vi "Configure.vi"(8 "error in":errorcluster, 10 "name":string, 11 "cPAS in":refnum<class "cPAS.lvclass">) -> (0 "error out":errorcluster, 3 "cPAS out":refnum<class "cPAS.lvclass">)   [LabVIEW 2015, in "cPAS.lvclass"]
doc: "Configure the Instrument object. The default behavior is to provide a name and define a command enqueuer."
uses:
  cPAS.lvclass
  Data/cPAS Data.lvclass
  Data/cPAS Cell Data/cPAS Cell Data.lvclass
  Reusable/PAS/Data/Main/Write CellData.vi
  Reusable/PAS/Main/Write Data.vi
  Reusable/PAS/Main/PAS.lvclass
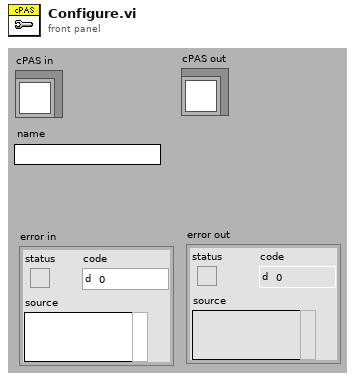
[diagram p1: front panel]
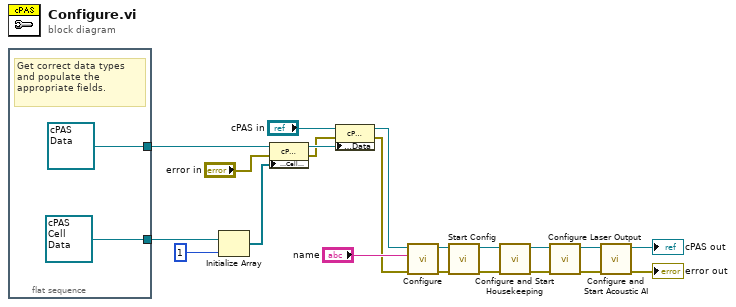
[diagram p0: block diagram]
diagram:
  n1 = flat-sequence {
    tunnel: [refnum<class "cPAS Data.lvclass"> refnum ("cPAS Data")] -> w10
    tunnel: [refnum<class "cPAS Cell Data.lvclass"> refnum ("cPAS Cell")] -> w9
    frame #0 {
      # "Get correct data types and populate the appropriate fields."
    }
  }
  n2 = Initialize Array(w9, 1 ("dimension size")) -> (w7:refnum<class "cPAS Cell Data.lvclass">[])
  n3 = property class="cPAS Data"(reference=w10, error in="error in", "Data Access:Cell Data"=w7) -> (reference out=w4:refnum<class "cPAS Data.lvclass">, error out=w2:errorcluster)
  n4 = property class="cPAS"(reference="cPAS in", error in=w2, "Data Access:Data"=w4) -> (reference out=w5:refnum<class "cPAS.lvclass">, error out=w1:errorcluster)
  n5 = call-parent "Configure.vi"("error in"=w1, "name"="name", "PAS in"=w5) -> ("error out"=w13:errorcluster, "PAS out"=w20:refnum<class "cPAS.lvclass">)  [unwired: 7 in]
  n6 = call-dynamic "Start Config.vi"("error in"=w13, "cPAS in"=w20) -> ("error out"=w18:errorcluster, "cPAS out"=w19:refnum<class "cPAS.lvclass">)  [unwired: 8 in]
  n7 = call-dynamic "Configure and Start Housekeeping.vi"("error in"=w18, "cPAS in"=w19) -> ("error out"=w16:errorcluster, "cPAS out"=w17:refnum<class "cPAS.lvclass">)  [unwired: 8 in]
  n8 = call-dynamic "Configure Laser Output.vi"("error in"=w16, "cPAS in"=w17) -> ("error out"=w14:errorcluster, "cPAS out"=w15:refnum<class "cPAS.lvclass">)  [unwired: 8 in]
  n9 = call-dynamic "Configure and Start Acoustic AI.vi"("error in"=w14, "cPAS in"=w15) -> ("error out"=→"error out":errorcluster, "cPAS out"=→"cPAS out":refnum<class "cPAS.lvclass">)  [unwired: 8 in]
